vi "Actor Core.vi"(8 "error in":errorcluster, 11 "Restaurant Manager UI in":refnum<class "Restaurant Manager UI.lvclass">) -> (0 "error out":errorcluster, 3 "Actor out":refnum<class "Actor.lvclass">)   [LabVIEW 2023, in "Restaurant Manager UI.lvlib" / "Restaurant Manager UI.lvclass"]
doc: "(<B>Filename</B>: Actor Framework.lvlib:Actor.lvclass:Actor Core.vi)\n\nReceives messages to the actor, reacts to them, and initiates any error handling that may shut the actor down.\n\nDescendant classes may override this VI to append parallel tasks for the actor to complete while it handles messages. Overrides use the Call Parent Class Method node."
uses:
  Restaurant Manager UI.lvclass
  C:/Users/bhaghyaraj/Trainings/NI Actor Framework/SDLC/UI Base/UI Base/UI Base.lvclass
  C:/Program Files/National Instruments/LabVIEW 2023/vi.lib/ActorFramework/Actor/Actor.lvclass
  <vilib>/ActorFramework/Actor/Actor.lvclass
  Restaurant Manager UI.lvclass/Restaurant Manager UI.ctl
  <vilib>/ActorFramework/Actor/Actor.lvclass/Actor.ctl
  <vilib>/ActorFramework/Message Enqueuer/Message Enqueuer.lvclass/Message Enqueuer.ctl
  <vilib>/ActorFramework/Message Enqueuer/Init from Existing Queue.vi
  <vilib>/ActorFramework/Message Enqueuer/Enqueue.vi
  <vilib>/ActorFramework/Stop Msg/Stop Msg.lvclass
  C:/Program Files/National Instruments/LabVIEW 2023/vi.lib/ActorFramework/Message/Message.lvclass
  <vilib>/ActorFramework/Message Priority Queue/Priority Enqueue.vi
  <vilib>/ActorFramework/Message Enqueuer/Message Enqueuer.lvclass
  UI Base/UI Base/UI Base.lvclass
panel:
  in  "Update Menu":bool
  in  "Move to Completed":bool
  in  "Move to Progress":bool
  in  "Create Order":bool
  out "Order Summary":string
  in  "Completed":i32(listbox)
  in  "In Progress":i32(listbox)
  in  "New Orders":i32(listbox)
  # "Restaurant Management"
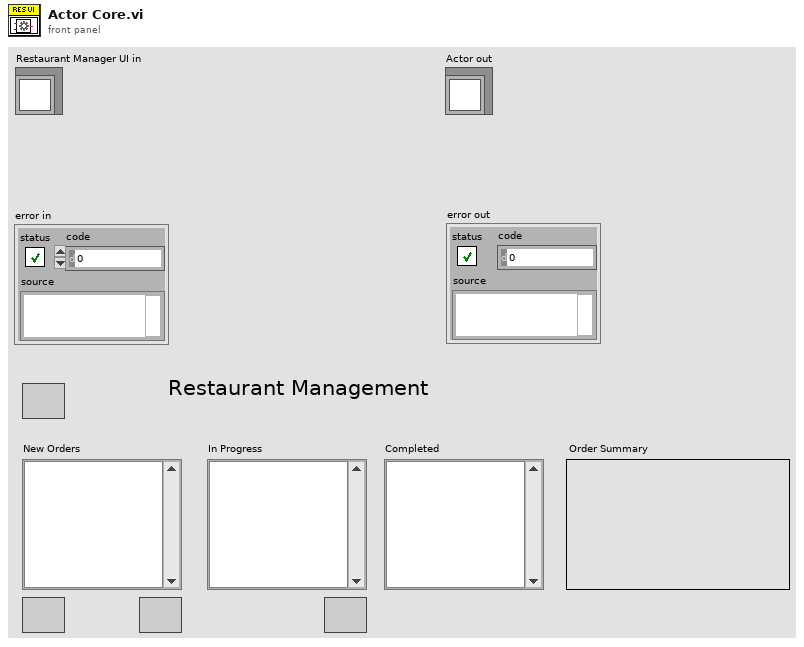
[diagram p1: front panel]
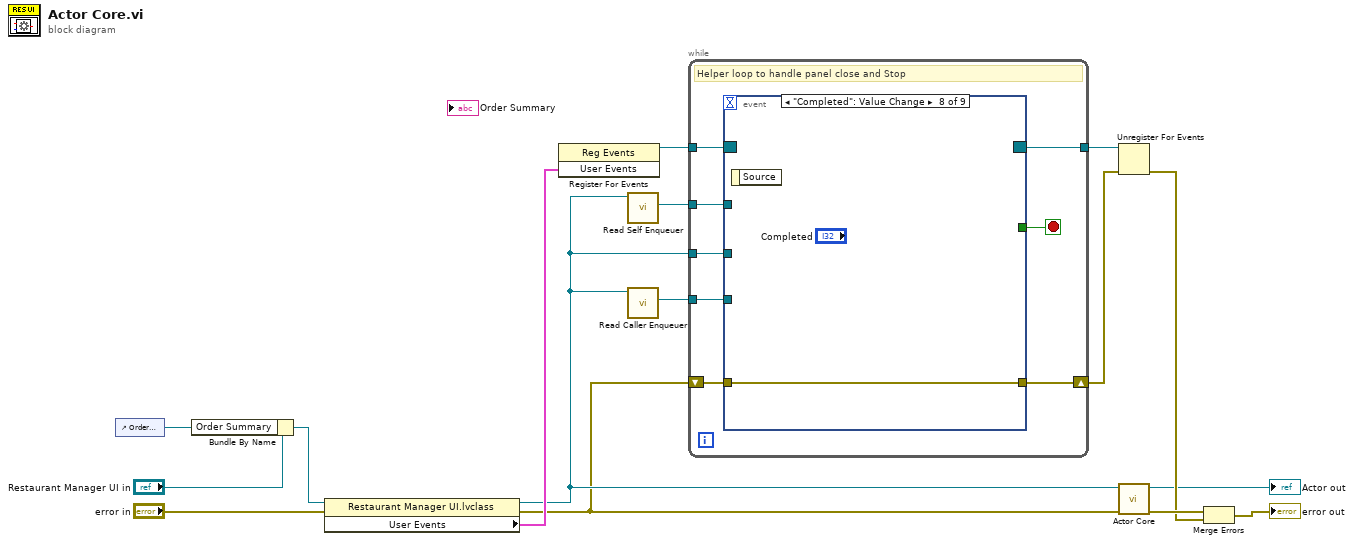
[diagram p0: block diagram]
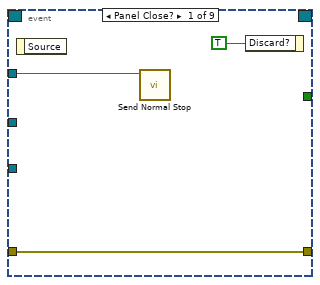
[diagram p2: hidden frame]
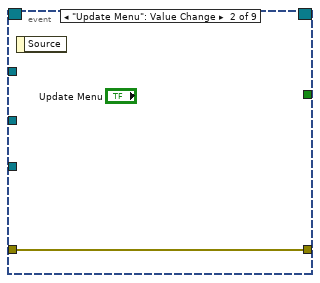
[diagram p3: hidden frame]
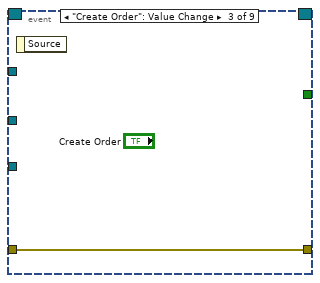
[diagram p4: hidden frame]
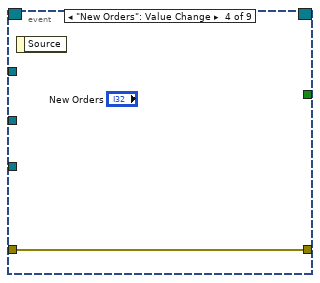
[diagram p5: hidden frame]
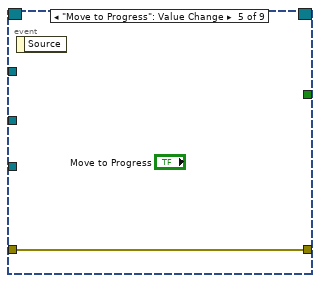
[diagram p6: hidden frame]
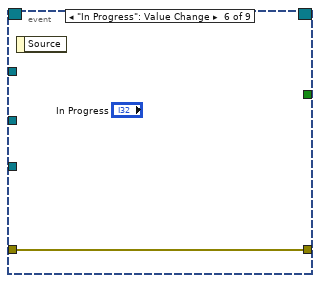
[diagram p7: hidden frame]
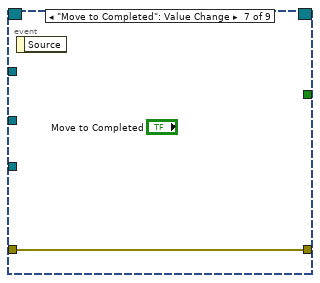
[diagram p8: hidden frame]
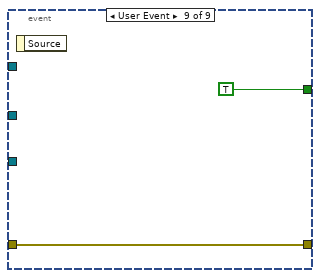
[diagram p9: hidden frame]
diagram:
  n1 = control-ref of="Order Summary"() -> (w3:refnum<vi>)
  n2 = Bundle By Name(cluster="Restaurant Manager UI in", "Order Summary"=w3) -> (w4:refnum<class "Restaurant Manager UI.lvclass">)
  n3 = property class="Restaurant Manager UI.lvclass"(reference=w4, error in="error in") -> (reference out=w9:refnum<class "Restaurant Manager UI.lvclass">, error out=w2:errorcluster, "User Events"=w12:cluster{"Stop":refnum<user-event>})
  n4 = register-events(w12) -> (reference out=w14:refnum<event-registration>)  [unwired: 2 in, 1 out]
  n5 = call <vilib>:"Read Self Enqueuer.vi"("Actor"=w9) -> ("Self Enqueuer"=w13:refnum<class "Message Enqueuer.lvclass">)  [unwired: 10 in]
  n6 = call <vilib>:"Read Caller Enqueuer.vi"("Actor"=w9) -> ("Caller Enqueuer"=w10:refnum<class "Message Enqueuer.lvclass">)  [unwired: 10 in]
  n7 = while {
    tunnel: w13 -> [w24]
    tunnel: w14 -> [w23]
    tunnel: [w21] -> w15
    tunnel: w10 -> [w20]
    tunnel: w9 -> [w19]
    shift-right: [w17] -> w1
    shift-left: w2 -> [w18]
    stop <- w22 stop-if-true
    # "Helper loop to handle panel close and Stop"
    n8 = event shown="[7] \"Completed\": Value Change" {
      selector: w23 -> [_ _ _ _ _ _ _ _ _]
      dyn-events: [_ _ _ _ _ _ _ _ _] -> w21
      timeout: _ -> [_ _ _ _ _ _ _ _ _]
      tunnel: w24 -> [w26 _ _ _ _ _ _ _ _]
      tunnel: [_ _ _ _ _ _ _ _ TRUE] -> w22
      tunnel: w20 -> [_ _ _ _ _ _ _ _ _]
      tunnel: w19 -> [_ _ _ _ _ _ _ _ _]
      tunnel: w18 -> [w25 w28 w29 w30 w31 w32 w33 w34 w35]
      tunnel: [w25 w28 w29 w30 w31 w32 w33 w34 w35] -> w17
      event Panel Close? {
        n9 = event-data() -> ()  [unwired: 1 in, 1 out]
        n10 = call <vilib>:"Send Normal Stop.vi"("Message Enqueuer"=w26) -> ()  [unwired: 10 in, 1 out]
        n11 = event-data("Discard?"=TRUE) -> ()  [unwired: 1 in, 1 out]
      }
      event "Update Menu": Value Change {
        n12 = event-data() -> ()  [unwired: 1 in, 1 out]
      }
      event "Create Order": Value Change {
        n13 = event-data() -> ()  [unwired: 1 in, 1 out]
      }
      event "New Orders": Value Change {
        n14 = event-data() -> ()  [unwired: 1 in, 1 out]
      }
      event "Move to Progress": Value Change {
        n15 = event-data() -> ()  [unwired: 1 in, 1 out]
      }
      event "In Progress": Value Change {
        n16 = event-data() -> ()  [unwired: 1 in, 1 out]
      }
      event "Move to Completed": Value Change {
        n17 = event-data() -> ()  [unwired: 1 in, 1 out]
      }
      event "Completed": Value Change {
        n18 = event-data() -> ()  [unwired: 1 in, 1 out]
      }
      event User Event {
        n19 = event-data() -> ()  [unwired: 1 in, 1 out]
      }
    }
  }
  n20 = Unregister For Events(event registration refnum=w15, error in=w1) -> (error out=w11:errorcluster)
  n21 = call-parent "Actor Core.vi"("error in"=w2, "Actor in"=w9) -> ("error out"=w16:errorcluster, "Actor out"=→"Actor out":refnum<class "Actor.lvclass">)  [unwired: 8 in]
  n22 = Merge Errors(w16, w11) -> (→"error out":errorcluster)
